vi "result file write data.vi"(8 "error in (no error)":errorcluster, 10 "raw data":T1, 11 "refnum":refnum<file>) -> (0 "error out":errorcluster, 3 "refnum out":refnum<file>)   [LabVIEW 2013]
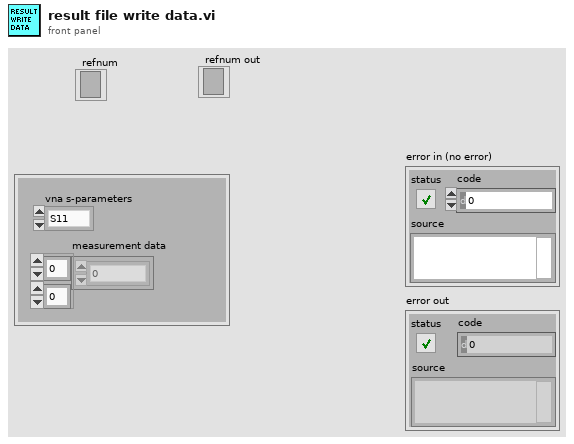
[diagram p1: front panel]
types:
  T1 = cluster{"measurement data":dbl[][], "vna s-parameters":enum16{"S11", "S12", "S21", "S22"}}
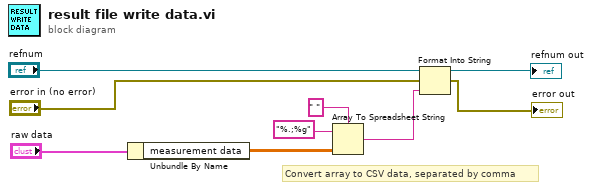
[diagram p0: block diagram]
diagram:
  # "Convert array to CSV data, separated by comma"
  n1 = Unbundle By Name("raw data") -> ("measurement data"=w1:dbl[][])
  n2 = Array To Spreadsheet String(delimiter (Tab)=" ", array=w1, 3:"%.;%g") -> (spreadsheet string=w6:string)
  n3 = Format Into String(initial string="refnum", error in="error in (no error)", w6) -> (resulting string=→"refnum out":refnum<file>, error out=→"error out":errorcluster)  [unwired: 1 in]
